vi "Read Digital Ouputs.vi"(8 "error in (no error)":errorcluster, 11 "PXI6521 in":refnum<class "PXI6521.lvclass">) -> (0 "error out":errorcluster, 2 "Digital Outputs Status":bool[](array[boolean]), 3 "PXI6521 out":refnum<class "PXI6521.lvclass">)   [LabVIEW 2018, in "PXI6521.lvlib" / "PXI6521.lvclass"]
uses:
  PXI6521.lvclass
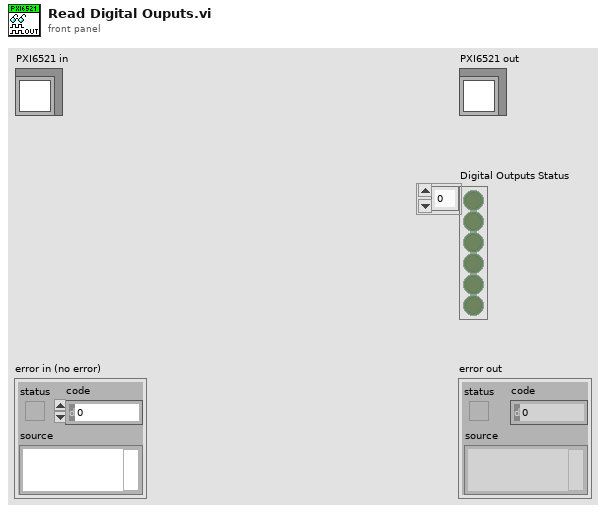
[diagram p1: front panel]
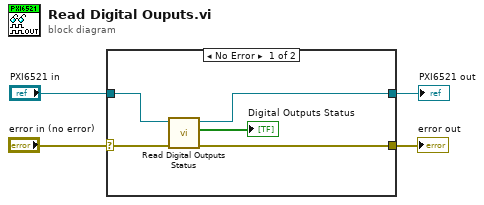
[diagram p0: block diagram]
diagram:
  n1 = case shown="No Error" "error in (no error)" {
    selector: "error in (no error)" -> [w9 w11]
    tunnel: [w7 w11] -> w3
    tunnel: [w6 w10] -> w1
    tunnel: "PXI6521 in" -> [w8 w10]
    frame No Error {
      n2 = call "Read Digital Outputs Status.vi"("error in (no error)"=w9, "PXI6521 in"=w8) -> ("error out"=w7:errorcluster, "Digital Outputs Status"=→"Digital Outputs Status":bool[], "PXI6521 out"=w6:refnum<class "PXI6521.lvclass">)  [unwired: 7 in]
    }
    frame Error {
    }
  }
  "error out" <- w3
  "PXI6521 out" <- w1
